vi "Graficadora1.vi"() -> ()   [LabVIEW 2020]
panel:
  out "Alarma":bool
  out "Waveform Chart":dynamicdata(graph)
  in  "Numeric":dbl
  in  "Slide":dbl(slide) scale=0.0..100.0
  in  "stop":bool
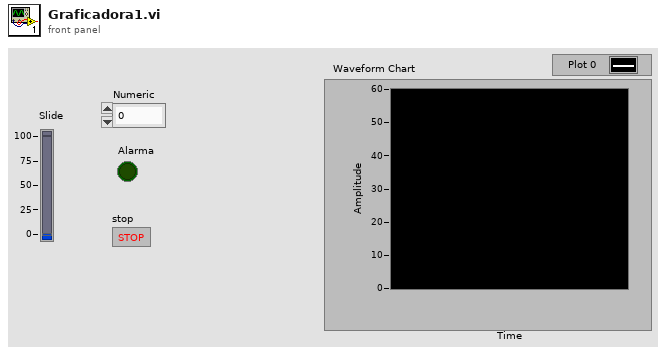
[diagram p1: front panel]
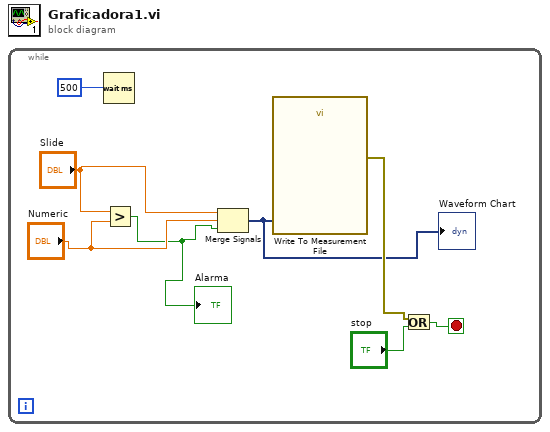
[diagram p0: block diagram]
diagram:
  n1 = while {
    stop <- w7 stop-if-true
    n2 = Wait (ms)(milliseconds to wait=500) -> ()  [unwired: 1 out]
    n3 = Greater?(x="Slide", y="Numeric") -> (0:w2:bool)
    "Alarma" <- w2
    n4 = Merge Signals("Slide", "Numeric", w2) -> (w1:dynamicdata)
    "Waveform Chart" <- w1
    n5 = call "Write To Measurement File"("Signals"=w1) -> ("error out"=w5:errorcluster)  [unwired: 16 in, 2 out]
    n6 = Or(x=w5, y="stop") -> (x .or. y?=w7:bool)
  }
